vi "GetDataInfo.vi"(8 "error in (no error)":errorcluster, 10 "Name":string, 11 "CarexMData in":refnum<class "ExpData.lvclass">) -> (0 "error out":errorcluster, 1 "Index":i8, 2 "Size":i8, 3 "CarexMData out":refnum<class "ExpData.lvclass">, 4 "ColHeaders":string[](array[string]))   [LabVIEW 2016, in "ExpData.lvclass"]
uses:
  ExpData.lvclass
  ExpData.lvclass/ExpData.ctl
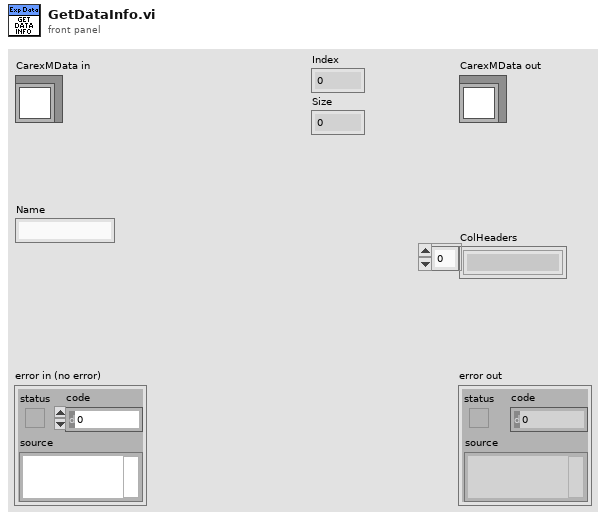
[diagram p1: front panel]
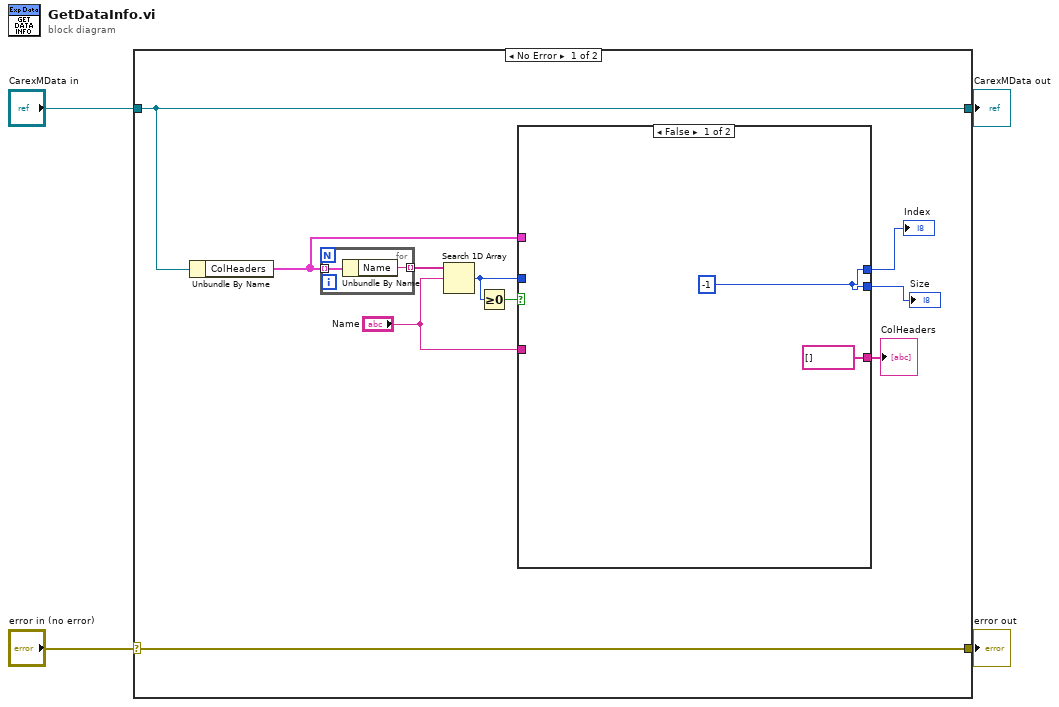
[diagram p0: block diagram]
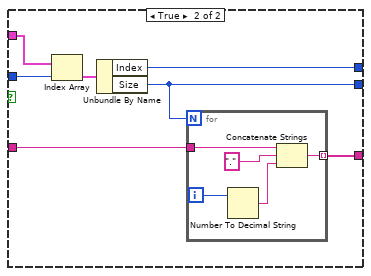
[diagram p2: hidden frame]
diagram:
  n1 = case shown="No Error" "error in (no error)" {
    selector: "error in (no error)" -> [w14 w32]
    tunnel: [w14 w32] -> w3
    tunnel: [w13 w31] -> w1
    tunnel: "CarexMData in" -> [w13 w31]
    frame No Error {
      n2 = Unbundle By Name(w13) -> ("ColHeaders"=w9:cluster{"Name":string, "Index":i8, "Size":i8}[])
      n3 = for {
        tunnel: w9 -> [w30] mode=indexing
        tunnel: [w29] -> w12 mode=indexing
        n4 = Unbundle By Name(w30) -> ("Name"=w29:string)
      }
      n5 = Search 1D Array(1D array=w12, element="Name") -> (index of element=w10:i32)  [unwired: 1 in]
      n6 = Greater Or Equal To 0?(x=w10) -> (x >= 0?=w11:bool)
      n7 = case shown="False" w11 {
        tunnel: w10 -> [_ w23]
        tunnel: w9 -> [_ w22]
        tunnel: "Name" -> [_ w20]
        tunnel: [string[] [] w19] -> w7
        tunnel: [w15 w18] -> w6
        tunnel: [w15 w17] -> w5
        frame False {
          w15 = -1
        }
        frame True {
          n8 = Index Array(array=w22, index=w23) -> (element=w21:cluster{"Name":string, "Index":i8, "Size":i8})
          n9 = Unbundle By Name(w21) -> ("Index"=w18:i8, "Size"=w17:i8)
          n10 = for {
            N: w17 -> [_]
            tunnel: w20 -> [w28]
            tunnel: [w24] -> w19 mode=indexing
            i -> [w26]
            n11 = Number To Decimal String(number=w26) -> (decimal integer string=w25:string)  [unwired: 1 in]
            n12 = Concatenate Strings(w28, "." ("string"), w25) -> (w24:string)
          }
        }
      }
      "ColHeaders" <- w7
      "Index" <- w6
      "Size" <- w5
    }
    frame Error {
    }
  }
  "error out" <- w3
  "CarexMData out" <- w1
